vi "Calculate And Update IMG.vi"(0 "pictuer_pupil_Original":string, 1 "pictuer_pupil_Processing":string, 2 "pictuer_WTW_Processing":string, 5 "pictuer_WTW_Original":string, 7 "D":dbl, 11 "error in (no error)":errorcluster caption="错误输入（无错误）", 12 "picture_Processing_K":string, 13 "picture_Processing_ALL":string) -> (4 "a":dbl, 6 "b":dbl, 8 "PD":dbl, 10 "WTW":dbl, 15 "error out":errorcluster caption="错误输出")   [LabVIEW 2015, in "Digital Image Processing.lvlib"]
doc: "该模板用于创建子VI。"
uses:
  Digital Image Processing.lvlib
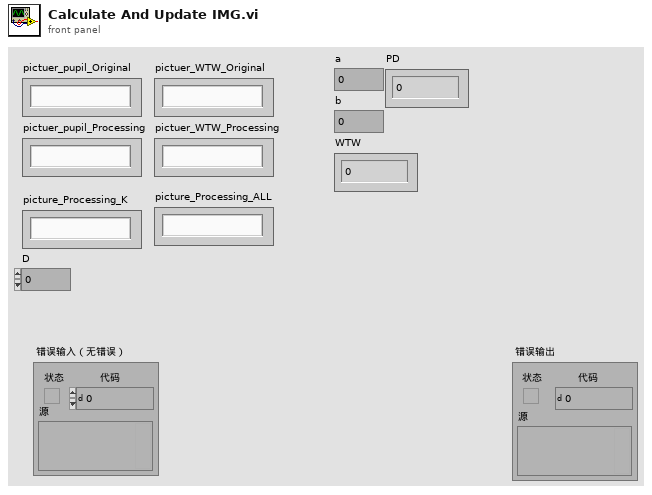
[diagram p1: front panel]
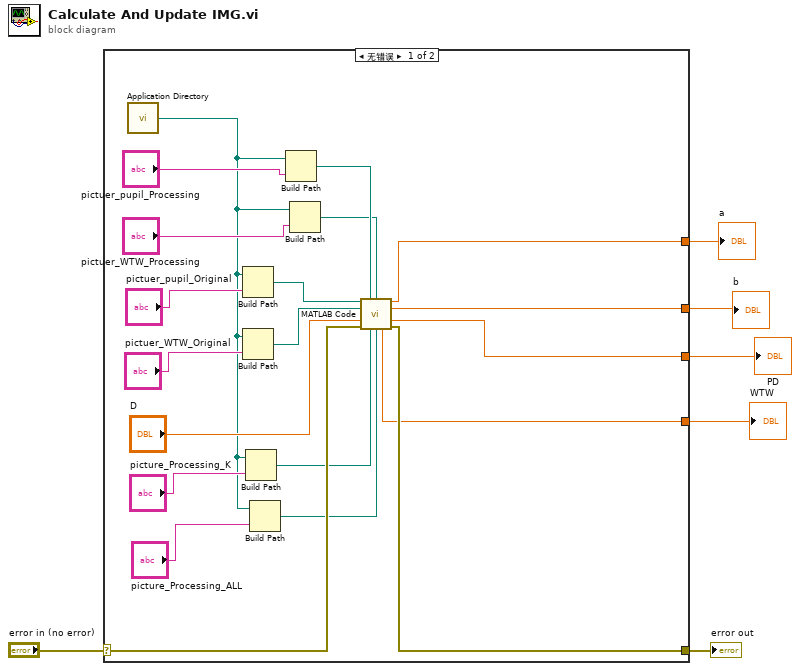
[diagram p0: block diagram]
diagram:
  n1 = case shown="无错误" "error in (no error)" {
    selector: "error in (no error)" -> [w21 w27]
    tunnel: [w11 w27] -> w5
    tunnel: [w10 _] -> w4
    tunnel: [w9 _] -> w3
    tunnel: [w8 _] -> w2
    tunnel: [w7 _] -> w1
    frame No Error {
      n2 = call <vilib>:"Application Directory.vi"() -> ("Application Directory"=w14:path)
      n3 = Build Path(base path=w14, name or relative path="pictuer_pupil_Original") -> (appended path=w24:path)
      n4 = Build Path(base path=w14, name or relative path="pictuer_WTW_Original") -> (appended path=w23:path)
      n5 = Build Path(base path=w14, name or relative path="picture_Processing_K") -> (appended path=w13:path)
      n6 = Build Path(base path=w14, name or relative path="picture_Processing_ALL") -> (appended path=w12:path)
      n7 = Build Path(base path=w14, name or relative path="pictuer_pupil_Processing") -> (appended path=w18:path)
      n8 = Build Path(base path=w14, name or relative path="pictuer_WTW_Processing") -> (appended path=w17:path)
      n9 = call "MATLAB Code.vi"("Path_IR"=w24, "PD_Process"=w18, "WTW_Process"=w17, "Path_WTW"=w23, "D"="D", "error in (no error)"=w21, "K_Process"=w13, "A_Process"=w12) -> ("a"=w10:dbl, "b"=w9:dbl, "PD"=w8:dbl, "WTW"=w7:dbl, "error out"=w11:errorcluster)  [unwired: 3 in]
    }
    frame Error {
    }
  }
  "error out" <- w5
  "a" <- w4
  "b" <- w3
  "PD" <- w2
  "WTW" <- w1
